vi "sort P(x) and q(x) by order (DBL).vi"(0 "p":dbl[](array[numeric]), 1 "q":dbl[](array[numeric])) -> (2 "high order polynomial":dbl[](array[numeric]), 3 "high order":i32, 4 "low order polynomial":dbl[](array[numeric]), 5 "low order":i32)   [LabVIEW 2020, in "NI_AALPro.lvlib"]
uses:
  <vilib>/Analysis/NI_AALPro.lvlib
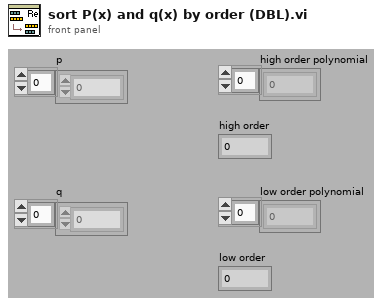
[diagram p1: front panel]
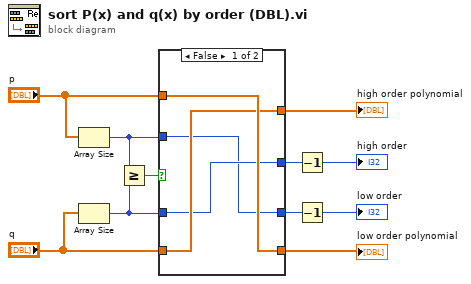
[diagram p0: block diagram]
diagram:
  n1 = Array Size(array="p") -> (size(s)=w10:i32)
  n2 = Array Size(array="q") -> (size(s)=w9:i32)
  n3 = Greater Or Equal?(x=w10, y=w9) -> (x >= y?=w11:bool)
  n4 = case shown="False" w11 {
    tunnel: "p" -> [w15 w19]
    tunnel: "q" -> [w14 w18]
    tunnel: [w15 w18] -> w3
    tunnel: [w14 w19] -> w6
    tunnel: w10 -> [w12 w17]
    tunnel: [w13 w17] -> w5
    tunnel: [w12 w16] -> w4
    tunnel: w9 -> [w13 w16]
    frame False {
    }
    frame True {
    }
  }
  "high order polynomial" <- w6
  "low order polynomial" <- w3
  n5 = Decrement(x=w5) -> (x-1=→"high order":i32)
  n6 = Decrement(x=w4) -> (x-1=→"low order":i32)
